vi "Enumerate Devices.vi"(8 "error in (no error)":errorcluster, 11 "HAL Editor in":refnum<class "HAL Editor.lvclass">) -> (0 "error out":errorcluster, 3 "HAL Editor out":refnum<class "HAL Editor.lvclass">)   [LabVIEW 2012, in "HAL Config.lvlib" / "HAL Editor.lvclass"]
uses:
  HAL Editor.lvclass
  build/ppl/lv-hal.lvlibp/Device/Device.lvclass
  <vilib>/Utility/LVLibp/NI_PackedLibraryUtility.lvlib
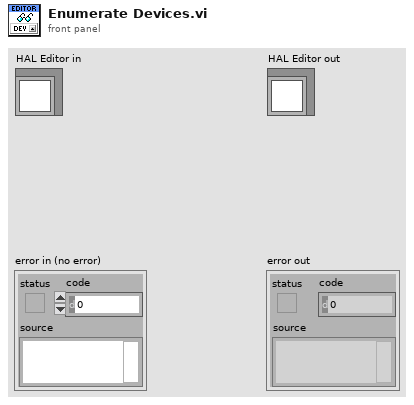
[diagram p1: front panel]
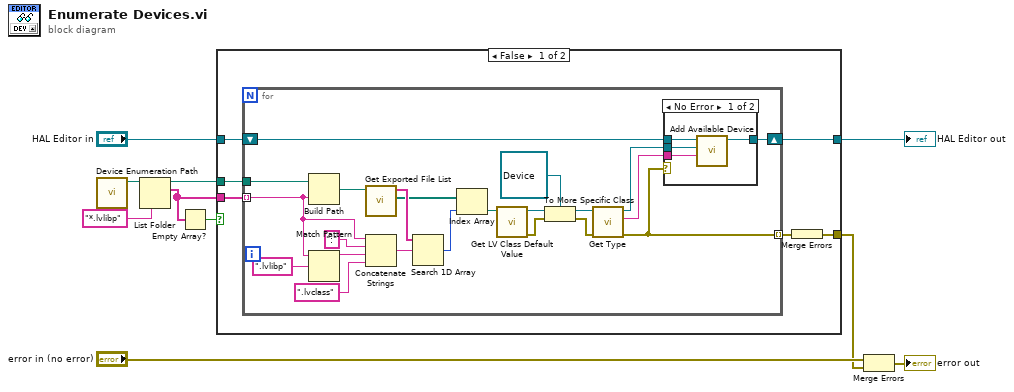
[diagram p0: block diagram]
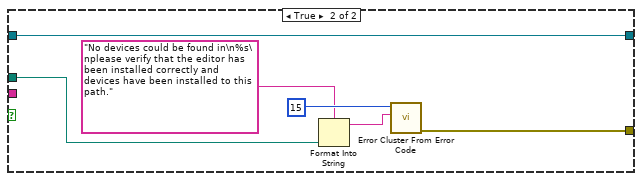
[diagram p3: hidden frame]
diagram:
  n1 = call "Device Enumeration Path.vi"() -> ("Device Enumeration Path"=w10:path)  [unwired: 11 in]
  n2 = List Folder(path=w10, pattern="*.lvlibp") -> (path out=w6:path, filenames=w3:string[])  [unwired: 2 in, 2 out]
  n3 = Empty Array?(array=w3) -> (empty?=w2:bool)
  n4 = case shown="False" w2 {
    tunnel: w6 -> [w16 w47]
    tunnel: "HAL Editor in" -> [w15 w44]
    tunnel: [w14 w44] -> w4
    tunnel: w3 -> [w13 _]
    tunnel: [w11 w45] -> w1
    frame False {
      n5 = for {
        tunnel: w13 -> [w17] mode=indexing
        tunnel: w16 -> [w35]
        shift-right: [w25] -> w14
        shift-left: w15 -> [w29]
        tunnel: [w26] -> w12 mode=indexing
        n6 = Build Path(base path=w35, name or relative path=w17) -> (appended path=w24:path)
        n7 = Match Pattern(string=w17, regular expression=".lvlibp") -> (before substring=w37:string)  [unwired: 1 in, 3 out]
        n8 = call <vilib>:"Get Exported File List.vi"("packed library path"=w24) -> ("paths"=w20:path[], "qualified names"=w21:string[])  [unwired: 8 in, 1 out]
        n9 = Concatenate Strings(w17, ":" ("string"), w37, ".lvclass" ("string")) -> (w22:string)
        n10 = Search 1D Array(1D array=w21, element=w22) -> (index of element=w19:i32)  [unwired: 1 in]
        n11 = Index Array(array=w20, index=w19) -> (element=w18:path)
        n12 = call <vilib>:"Get LV Class Default Value.vi"("class path"=w18) -> ("error out"=w31:errorcluster, "object"=w34:refnum<class>)  [unwired: 9 in]
        n13 = To More Specific Class(target class=refnum<class "Device.lvclass"> refnum ("lv-hal.lvlibp:Device.lvclass"), reference=w34, error in=w31) -> (specific class reference=w32:refnum<class "Device.lvclass">, error out=w30:errorcluster)
        n14 = call-dynamic "Get Type.vi"("error in (no error)"=w30, "Device in"=w32) -> ("error out"=w26:errorcluster, "Type"=w28:string, "Device out"=w27:refnum<class "Device.lvclass">)  [unwired: 7 in]
        n15 = case shown="No Error" w26 {
          tunnel: w29 -> [w42 w43]
          tunnel: w28 -> [w41 _]
          tunnel: w27 -> [w40 _]
          tunnel: [w39 w43] -> w25
          frame No Error {
            n16 = call "Add Available Device.vi"("Type"=w41, "Device"=w40, "HAL Editor in"=w42) -> ("HAL Editor out"=w39:refnum<class "HAL Editor.lvclass">)  [unwired: 7 in, 1 out]
          }
          frame Error {
          }
        }
      }
      n17 = Merge Errors(w12) -> (w11:errorcluster)
    }
    frame True {
      n18 = Format Into String(format string="No devices could be found in\n%s\nplease verify that the editor has been installed correctly and devices have been installed to this path." ("error message (\"\")"), w47) -> (resulting string=w46:string)  [unwired: 2 in, 1 out]
      n19 = call <vilib>:"Error Cluster From Error Code.vi"("error message (\"\")"=w46, "error code (0)"=15) -> ("error out"=w45:errorcluster)  [unwired: 7 in]
    }
  }
  "HAL Editor out" <- w4
  n20 = Merge Errors("error in (no error)", w1) -> (→"error out":errorcluster)
